vi "UTL_JL_Calculate Final Value.vi"(8 "Error":errorcluster, 10 "Voltage Scalling":T1, 11 "Analog Value":dbl) -> (0 "Error Out":errorcluster, 3 "Analog Value Out":dbl)   [LabVIEW 2023]
doc: "Takes the scaling parameters and calculates final value."
uses:
  Controls/Cluster_JL Scaling Control.ctl
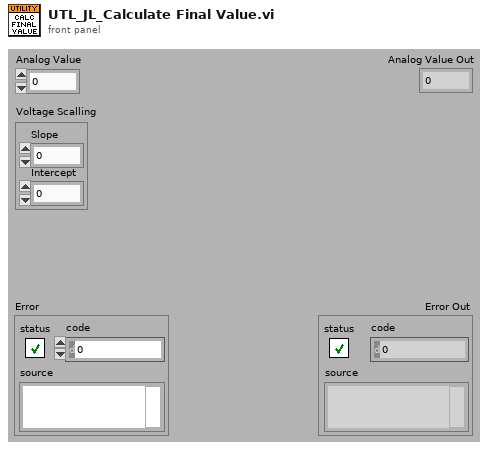
[diagram p1: front panel]
types:
  T1 = typedef "Cluster_JL Scaling Control.ctl" = cluster{"Slope":dbl, "Intercept":dbl}
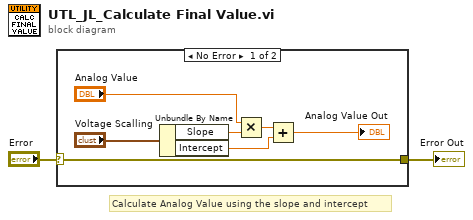
[diagram p0: block diagram]
diagram:
  # "Calculate Analog Value using the slope and intercept"
  n1 = case shown="No Error" "Error" {
    selector: "Error" -> [w9 w10]
    tunnel: [w9 w10] -> w1
    frame No Error {
      n2 = Unbundle By Name("Voltage Scalling") -> ("Slope"=w5:dbl, "Intercept"=w4:dbl)
      n3 = Multiply(x="Analog Value", y=w5) -> (x*y=w7:dbl)
      n4 = Add(x=w7, y=w4) -> (x+y=→"Analog Value Out":dbl)
    }
    frame Error {
    }
  }
  "Error Out" <- w1
